vi "WM Paddle Calibration.vi"(2 "Input Voltage":dbl[](array[numeric]) format="%.2f", 3 "Stroke Calibration (V/m)":dbl=7.8564 format="%.4f", 4 "Max 1/2 Piston Stroke (m)":dbl=0.16 format="%.2f", 5 "Input Stroke Distance (m)":dbl[](array[numeric]) format="%.2f") -> (0 "Output Stroke Distance":dbl[](array[numeric]) format="%.2f", 1 "Output Voltage":dbl[](array[numeric]) min=-2.0 max=2.0 format="%.2f")   [LabVIEW 2012]
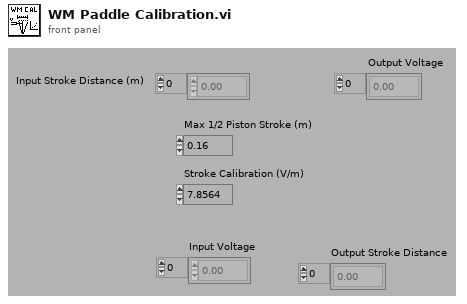
[diagram p1: front panel]
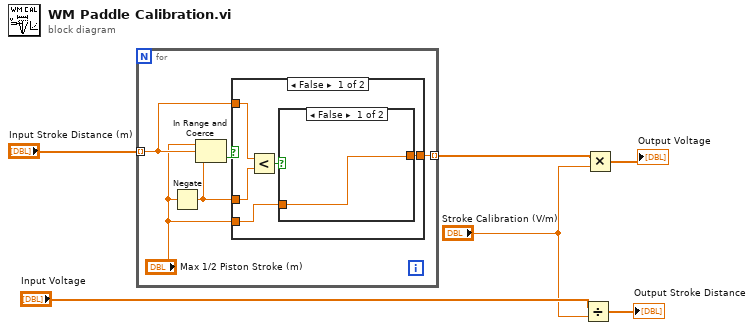
[diagram p0: block diagram]
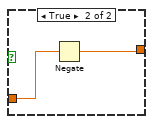
[diagram p2: hidden frame]
diagram:
  n1 = for {
    tunnel: "Input Stroke Distance (m)" -> [w9] mode=indexing
    tunnel: [w10] -> w3 mode=indexing
    n2 = Negate(x="Max 1/2 Piston Stroke (m)") -> (-x=w8:dbl)
    n3 = In Range and Coerce(upper limit="Max 1/2 Piston Stroke (m)", x=w9, lower limit=w8) -> (In Range?=w11:bool)  [unwired: 1 out]
    n4 = case shown="False" w11 {
      tunnel: [w13 w20] -> w10
      tunnel: w9 -> [w15 w20]
      tunnel: w8 -> [w16 _]
      tunnel: "Max 1/2 Piston Stroke (m)" -> [w12 _]
      frame False {
        n5 = Less?(x=w15, y=w16) -> (x < y?=w14:bool)
        n6 = case shown="False" w14 {
          tunnel: [w17 w18] -> w13
          tunnel: w12 -> [w17 w19]
          frame False {
          }
          frame True {
            n7 = Negate(x=w19) -> (-x=w18:dbl)
          }
        }
      }
      frame True {
      }
    }
  }
  n8 = Divide(x="Input Voltage", y="Stroke Calibration (V/m)") -> (x/y=→"Output Stroke Distance":dbl[])
  n9 = Multiply(x=w3, y="Stroke Calibration (V/m)") -> (x*y=→"Output Voltage":dbl[])
